vi "scripting function .vi"() -> ()   [LabVIEW 2020]
uses:
  <vilib>/numeric/LVNumericRepresentation.ctl
panel:
  out "error out 2":errorcluster
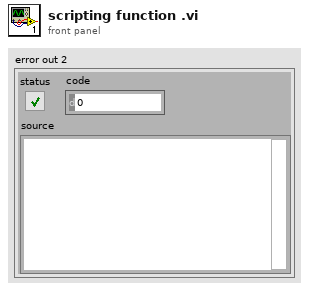
[diagram p1: front panel]
types:
  T1 = typedef "LVNumericRepresentation.ctl" = enum32{"Extended Precision", "Double Precision", "Single Precision", "Long", "Word", "Byte", "Unsigned Long", "Unsigned Word", "Unsigned Byte", "Complex Extended", "Complex Double", "Complex Single", "Quad", "Unsigned Quad", "Fixed-Point"}
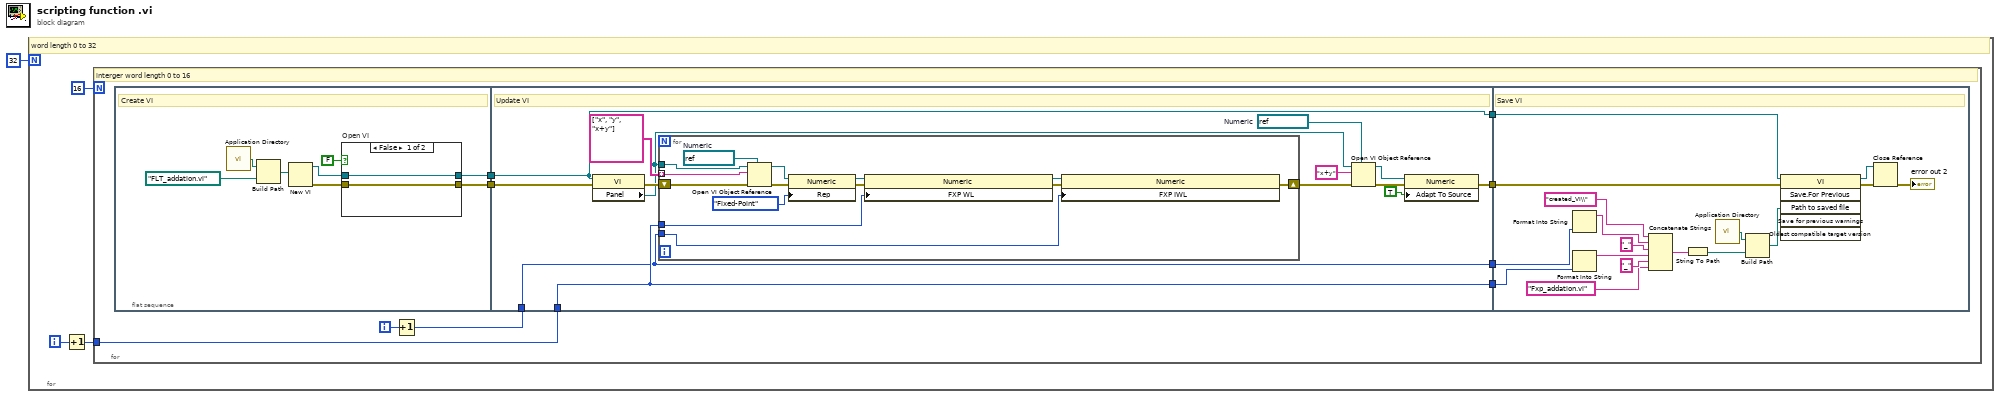
[diagram p0: block diagram]
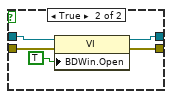
[diagram p2: hidden frame]
diagram:
  n1 = for {
    N: 32 -> [_]
    i -> [w4]
    # "word length 0 to 32"
    n2 = Increment(x=w4) -> (x+1=w2:i32)
    n3 = for {
      N: 16 -> [_]
      tunnel: w2 -> [w7]
      i -> [w6]
      # "interger word length 0 to 16"
      n4 = flat-sequence {
        tunnel: [w14] -> w13
        tunnel: [w15] -> w12
        tunnel: w5 -> [w30]
        tunnel: w7 -> [w31]
        tunnel: w13 -> [w29]
        tunnel: w12 -> [w40]
        tunnel: [w33] -> w11
        tunnel: [w31] -> w10
        tunnel: [w30] -> w9
        tunnel: [w29] -> w8
        tunnel: w11 -> [w61]
        tunnel: w10 -> [w59]
        tunnel: w9 -> [w58]
        tunnel: w8 -> [w57]
        frame #0 {
          # "Create VI"
          n5 = call <vilib>:"Application Directory.vi"() -> ("Application Directory"=w20:path)
          n6 = Build Path(base path=w20, name or relative path=path "FLT_addation.vi" ("vi path")) -> (appended path=w21:path)
          n7 = New VI(10:w21) -> (0:w19:errorcluster, 3:w18:refnum<vi>)  [unwired: 6 in]
          n8 = case "Open VI" shown="False" FALSE {
            tunnel: w18 -> [w22 w28]
            tunnel: w19 -> [w23 w27]
            tunnel: [w22 w25] -> w14
            tunnel: [w23 w24] -> w15
            frame False {
            }
            frame True {
              n9 = property class="VI"(reference=w28, error in=w27, "BDWin.Open"=TRUE ("Block Diagram Window:Open")) -> (reference out=w25:refnum<vi>, error out=w24:errorcluster)
            }
          }
        }
        frame #1 {
          w36 = refnum<vi> refnum  # Numeric
          # "Update VI"
          n10 = property on="Property Node" class="VI"(reference=w29, error in=w40) -> (error out=w42:errorcluster, "Panel"=w38:refnum<vi>)  [unwired: 1 out]
          n11 = for {
            tunnel: w38 -> [w54]
            tunnel: w30 -> [w50]
            tunnel: w31 -> [w49]
            shift-right: [w44] -> w39
            shift-left: w42 -> [w52]
            tunnel: string[] ["x", "y", "x+y"] -> [w48] mode=indexing
            w56 = refnum<vi> refnum  # Numeric
            n12 = Open VI Object Reference(7:w56, 8:w52, 10:w48, 11:w54) -> (0:w53:errorcluster, 3:w55:refnum<vi>)
            n13 = property on="Property Node" class="Numeric"(reference=w55, error in=w53, "Rep"=LVNumericRepresentation."Fixed-Point" ("new representation")) -> (reference out=w47:refnum<vi>, error out=w46:errorcluster)
            n14 = property on="Property Node" class="Numeric"(reference=w47, error in=w46, "FXP WL"=w49) -> (reference out=w43:refnum<vi>, error out=w45:errorcluster)
            n15 = property on="Property Node" class="Numeric"(reference=w43, error in=w45, "FXP IWL"=w50) -> (error out=w44:errorcluster)  [unwired: 1 out]
          }
          n16 = Open VI Object Reference(7:w36, 8:w39, 10:"x+y" ("name/order"), 11:w38) -> (0:w34:errorcluster, 3:w35:refnum<vi>)
          n17 = property on="Property Node" class="Numeric"(reference=w35, error in=w34, "Adapt To Source"=TRUE) -> (error out=w33:errorcluster)  [unwired: 1 out]
        }
        frame #2 {
          # "Save VI"
          n18 = Format Into String(w58) -> (resulting string=w71:string)  [unwired: 3 in, 1 out]
          n19 = Format Into String(w59) -> (resulting string=w72:string)  [unwired: 3 in, 1 out]
          n20 = Concatenate Strings("created_VI\\" ("string"), w71, "_" ("string"), w72, "_" ("string"), "Fxp_addation.vi" ("string")) -> (w60:string)
          n21 = String To Path(string=w60) -> (path=w73:path)
          n22 = call <vilib>:"Application Directory.vi"() -> ("Application Directory"=w69:path)
          n23 = Build Path(base path=w69, name or relative path=w73) -> (appended path=w70:path)
          n24 = invoke class="VI" method="Save.For Previous"(reference=w57, error in=w61, "Path to saved file"=w70) -> (reference out=w66:refnum<vi>, error out=w67:errorcluster)  [unwired: 3 in, 4 out]
          n25 = Close Reference(reference=w66, error in (no error)=w67) -> (error out=→"error out 2":errorcluster)
        }
      }
      n26 = Increment(x=w6) -> (x+1=w5:i32)
    }
  }
